vi "Read 200s Buffer.vi"(8 "error in":errorcluster, 11 "CPC in":refnum<class "3022A.lvclass">) -> (0 "error out":errorcluster, 2 "Counts":u32, 3 "CPC out":refnum<class "3022A.lvclass">)   [LabVIEW 2014, in "3022A.lvclass"]
uses:
  3022A/3022A.lvclass
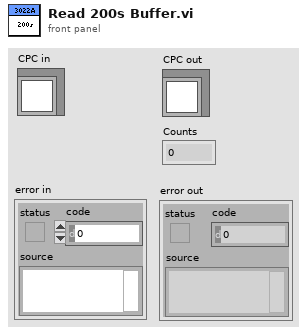
[diagram p1: front panel]
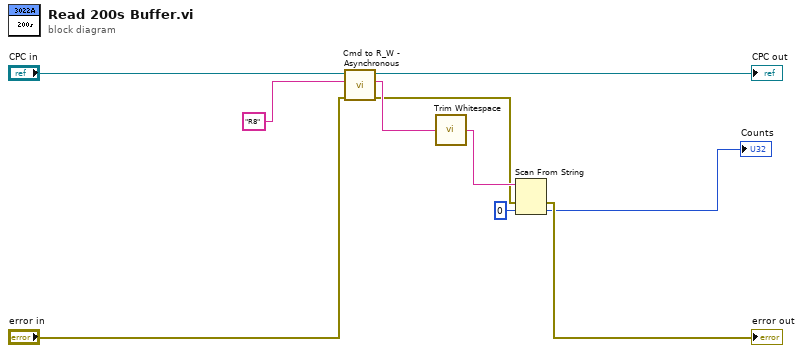
[diagram p0: block diagram]
diagram:
  n1 = call-dynamic "Cmd to R_W - Asynchronous.vi"("error in"="error in", "write buffer"="R8" ("string"), "Serial IO in"="CPC in") -> ("error out"=w1:errorcluster, "read buffer"=w4:string, "Serial IO out"=→"CPC out":refnum<class "3022A.lvclass">)  [unwired: 6 in]
  n2 = call <vilib>:"Trim Whitespace.vi"("string"=w4) -> ("trimmed string"=w3:string)  [unwired: 1 in]
  n3 = Scan From String(input string=w3, error in=w1, default 1=u32 0 ("default value 1")) -> (error out=→"error out":errorcluster, output 1=→"Counts":u32)  [unwired: 2 in, 2 out]
